vi "Embedded Progress Bar Q.vi"(2 "Progress Bar Queue Name":string="AlliGator Progress Bar Q") -> (6 "Progress Bar Queue":refnum<queue>)   [LabVIEW 2021, in "GUI.lvlib"]
uses:
  Embedded Progress Bar Q Element.ctl
  GUI.lvlib
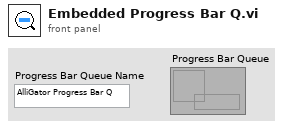
[diagram p1: front panel]
types:
  T1 = typedef "GUI.lvlib/Embedded Progress Bar Q Element.ctl" = cluster{"Action":string, "Value":dbl}
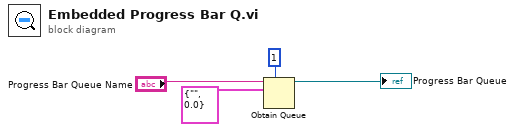
[diagram p0: block diagram]
diagram:
  n1 = Obtain Queue(max queue size (-1, unlimited)=1, name (unnamed)="Progress Bar Queue Name", element data type=T1 {"Action"="", "Value"=0.0}) -> (queue out=→"Progress Bar Queue":refnum<queue>)  [unwired: 2 in, 2 out]
